vi "MAX31855 Thermocouple Sensor.vi"   [LabVIEW 2014]
doc: "This example shows how to read temp data from MAX31888 sensor ."
uses:
  QwaveSys_Interface/QwaveSys_Interface.lvlib
  PWS_ESP8266/PWS_ESP8266.lvlib
panel:
  # "Overview: Demonstrates how to read Pmod TC-1 (MAX31855) Thermocouple sensor connected to digital pin.\nRequirements: LabVIEW Full Development System,Arduino Compatible Compiler for LabVIEW,Programmable Wireless Stamp (PWS) Library.\nInstructions:\n1. Plug-in thermocouple sensor MAX31855 module (Pmod TC-1) to SPI port refer diagram below.\n2.  If this example has been loaded from the Arduino Compatible Compiler for LabVIEW, simply select Compile and Download.  Otherwise, open Tools>Arduino Compatible Compiler for LabVIEW in LabVIEW, then select File>Load VI, and select this VI and then Compile and Download.\n3. Open \"Serial Monitor\" by select \"Tools>Serial Monitor\" and select baud rate to 9600.\n4. Observe the logged data being print out on serial port monitor."
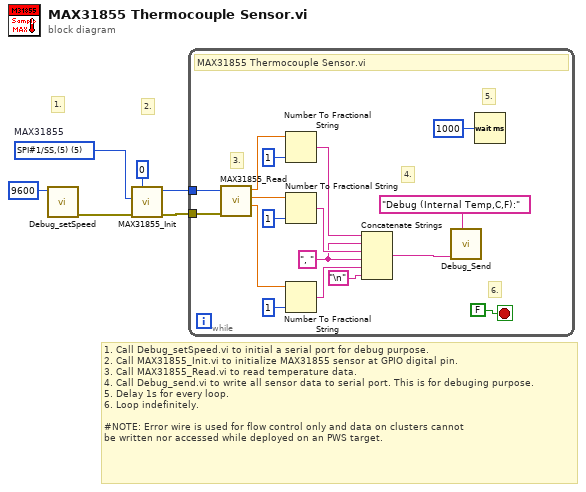
[diagram p0: block diagram]
diagram:
  w1 = u8 5 items=["SPI#1/SS,(5)"=5, "SPI#2/MOSI,(13)"=13, "SPI#3/MISO,(12)"=12, "SPI#4/SCLK,(14)"=14, "UART#1/CS,(15)"=15, "UART#2/TXD,(1)"=1, "UART#3/RXD,(3)"=3, "UART#4/LED,(16)"=16, "FPROM_Btn,(0)"=0, "SDCard_CS,(4)"=4, "I2C-SDA/TXD1,(2)"=2, "ADC0,(17)"=17]  # MAX31855
  # "1. Call Debug_setSpeed.vi to initial a serial port for debug purpose.\n2. Call MAX31855_Init.vi to initialize MAX31855 sensor at GPIO digital pin. \n3. Call MAX31855_Read.vi to read temperature data.\n4. Call Debug_send.vi to write all sensor data to serial port. This is for debuging purpose.\n5. Delay 1s for every loop.\n6. Loop indefinitely.\n\n#NOTE: Error wire is used for flow control only and data on clusters cannot\nbe written nor accessed while deployed on an PWS target."
  # "2."
  # "1."
  n1 = call "Debug_setSpeed.vi"("Speed"=u32 9600) -> ("error out"=w4:errorcluster)  [unwired: 10 in]
  n2 = call "MAX31855_Init.vi"("error in"=w4, "CS"=w1, "Interface (0-4)"=u8 0) -> ("error out"=w6:errorcluster, "Instance"=w5:u8)  [unwired: 7 in]
  n3 = while {
    tunnel: w6 -> [w23]
    tunnel: w5 -> [w9]
    stop <- FALSE stop-if-true
    w11 = ", " ("string")
    # "6."
    # "5."
    # "4."
    # "3."
    # "MAX31855 Thermocouple Sensor.vi"
    n4 = call "MAX31855_Read.vi"("Instance"=w9, "error in (no error)"=w23) -> ("Farenheit"=w13:dbl, "Celsius"=w20:dbl, "Internal Temp"=w21:dbl)  [unwired: 6 in, 1 out]
    n5 = Number To Fractional String(number=w21, precision (6)=i16 1) -> (F-format string=w19:string)  [unwired: 2 in]
    n6 = Number To Fractional String(number=w20, precision (6)=i16 1) -> (F-format string=w18:string)  [unwired: 2 in]
    n7 = Number To Fractional String(number=w13, precision (6)=i16 1) -> (F-format string=w10:string)  [unwired: 2 in]
    n8 = Concatenate Strings(w19, w11, w18, w11, w10, "\n" ("Line Feed Constant")) -> (w8:string)
    n9 = call "Debug_Send.vi"("Name"="Debug (Internal Temp,C,F):", "DATA"=w8) -> ()  [unwired: 10 in]
    n10 = Wait (ms)(milliseconds to wait=u32 1000) -> ()  [unwired: 1 out]
  }
